vi "PROG 1 - Writing Hello World.vi"() -> ()   [LabVIEW 2012]
panel:
  out "String":string
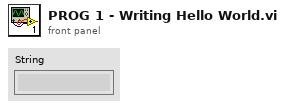
[diagram p1: front panel]
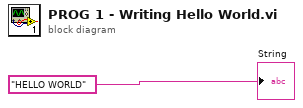
[diagram p0: block diagram]
diagram:
  "String" <- "HELLO WORLD"
